vi "POSTRequest.vi"(6 "expected response":T1=200 items=["200 OK"=200, "201 Created"=201, "400 Bad Request"=400, "401 Unauthorized"=401, "403 Forbidden"=403, "404 Not Found"=404, "405 Method Not Allowed"=405, "406 Not Acceptable"=406, "500 Internal Server Error"=500], 7 "Body in":string, 8 "error in (no error)":errorcluster, 9 "Parameter":string, 10 "Request":string, 11 "ByteRESTBase in":refnum<class "RESTBase.lvclass">) -> (0 "error out":errorcluster, 1 "Headers":string, 2 "Body":string, 3 "ByteRESTBase out":refnum<class "RESTBase.lvclass">)   [LabVIEW 2019, in "ByteREST.lvlib" / "RESTBase.lvclass"]
doc: "Effettua una richiesta di GET al server come:\nSERVER/api/bytegs/RICHIESTA/PARAMETRO(opzionale)"
uses:
  RESTBase.lvclass
  Status_Code.ctl
  RESTBase.lvclass/RESTBase.ctl
  <vilib>/httpClient/POSTBuffer.vi
  <vilib>/httpClient/LabVIEWHTTPClient.lvlib
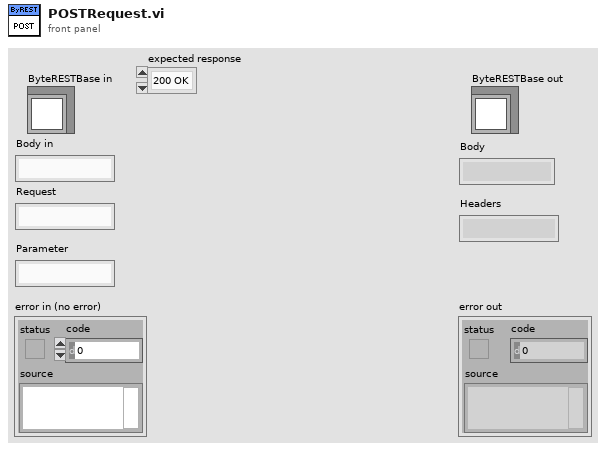
[diagram p1: front panel]
types:
  T1 = typedef "ByteREST.lvlib/RESTBase.lvclass/Status_Code.ctl" = u16
  T2 = typedef "LabVIEWHTTPClient.lvlib/ClientHandle.ctl" = refnum<k1>
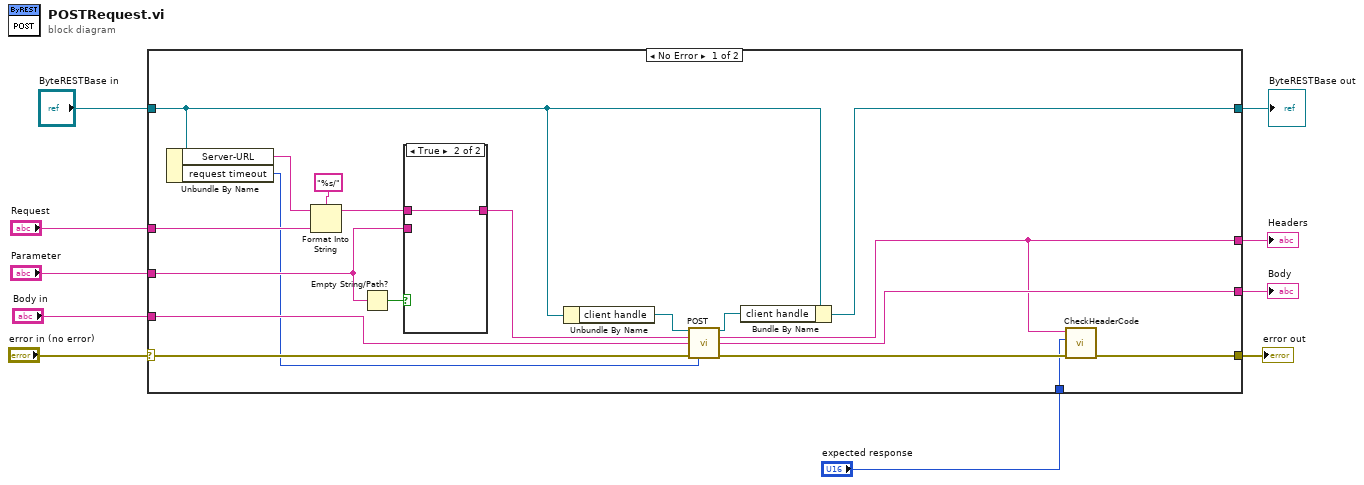
[diagram p0: block diagram]
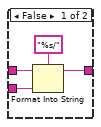
[diagram p2: hidden frame]
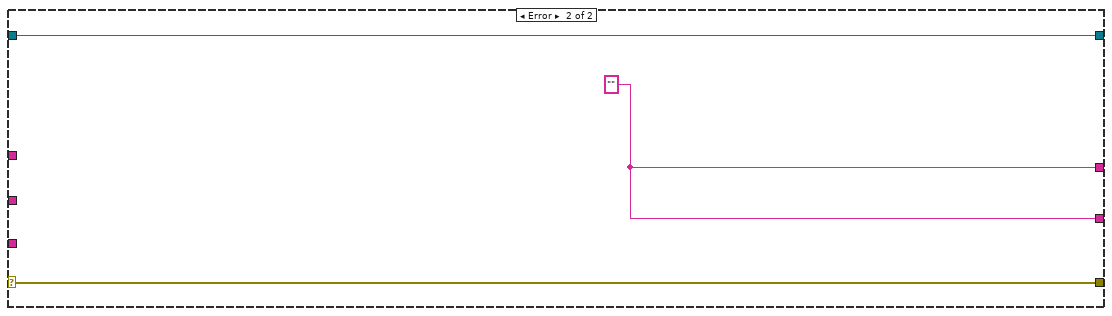
[diagram p3: hidden frame]
diagram:
  n1 = case shown="No Error" "error in (no error)" {
    selector: "error in (no error)" -> [w25 w37]
    tunnel: [w14 w37] -> w9
    tunnel: [w22 w36] -> w3
    tunnel: "ByteRESTBase in" -> [w19 w36]
    tunnel: "Request" -> [w17 _]
    tunnel: "Parameter" -> [w26 _]
    tunnel: [w21 w35] -> w6
    tunnel: [w15 w35] -> w5
    tunnel: "Body in" -> [w13 _]
    tunnel: "expected response" -> [w12 _]
    frame No Error {
      n2 = Unbundle By Name(w19) -> ("Server-URL"=w18:string, "request timeout"=w11:i32)
      n3 = Format Into String(format string="%s/" ("url"), initial string=w18, w17) -> (resulting string=w28:string)  [unwired: 1 in, 1 out]
      n4 = Empty String/Path?(string/path=w26) -> (empty?=w27:bool)
      n5 = case shown="True" w27 {
        tunnel: w28 -> [w32 w34]
        tunnel: [w30 w34] -> w24
        tunnel: w26 -> [w31 _]
        frame False {
          n6 = Format Into String(format string="%s/" ("url"), initial string=w32, w31) -> (resulting string=w30:string)  [unwired: 1 in, 1 out]
        }
        frame True {
        }
      }
      n7 = Unbundle By Name(w19) -> ("client handle"=w23:T2)
      n8 = call-poly <vilib>:"POST.vi"("client handle"=w23, "url"=w24, "buffer"=w13, "error in (no error)"=w25, "timeout (10000)"=w11) -> ("client handle out"=w20:T2, "headers"=w15:string, "body"=w21:string, "error out"=w16:errorcluster)  [unwired: 7 in]
      n9 = Bundle By Name(cluster=w19, "client handle"=w20) -> (w22:refnum<class "RESTBase.lvclass">)
      n10 = call "CheckHeaderCode.vi"("error in (no error)"=w16, "Expected code (200)"=w12, "Headers"=w15) -> ("error out"=w14:errorcluster)  [unwired: 8 in]
    }
    frame Error {
      w35 = "" ("body")
    }
  }
  "error out" <- w9
  "Body" <- w6
  "Headers" <- w5
  "ByteRESTBase out" <- w3
